vi "Create Priority Key.vi"(8 "Handler In":refnum<class "Handler.lvclass">, 11 "Index In":u16) -> (3 "Next Index":u16, 5 "Handler":refnum<class "Handler.lvclass">, 7 "Priority Key":T1)   [LabVIEW 2020, in "HTTP Server.lvlib" / "Server.lvclass"]
uses:
  Server.lvclass
  Priority.ctl
  HTTP Server.lvlib
  Handler/Handler.lvclass
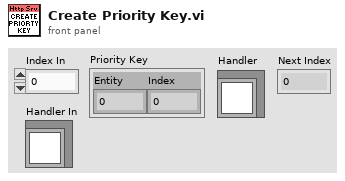
[diagram p1: front panel]
types:
  T1 = typedef "HTTP Server.lvlib/Priority.ctl" = cluster{"Entity":u16, "Index":u16}
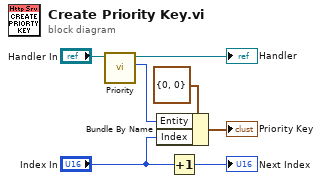
[diagram p0: block diagram]
diagram:
  n1 = call-dynamic "Priority.vi"("Handler in"="Handler In") -> ("Priority"=w6:u16, "Handler out"=→"Handler":refnum<class "Handler.lvclass">)  [unwired: 8 in, 1 out]
  n2 = Bundle By Name(cluster=T1 {"Entity"=0, "Index"=0} ("Priority"), "Entity"=w6, "Index"="Index In") -> (→"Priority Key":T1)
  n3 = Increment(x="Index In") -> (x+1=→"Next Index":u16)
